vi "ERROR_TEST_MESSAGE.vi"(8 "error in":errorcluster) -> (0 "error out":errorcluster)   [LabVIEW 2012]
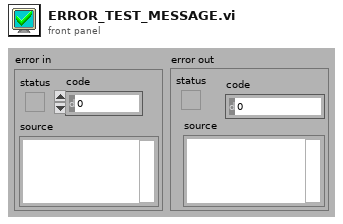
[diagram p1: front panel]
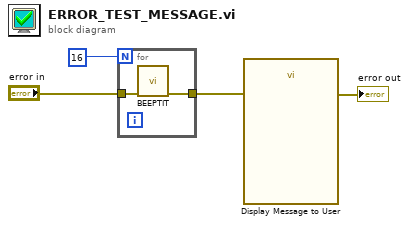
[diagram p0: block diagram]
diagram:
  n1 = for {
    N: 16 -> [_]
    tunnel: "error in" -> [w6]
    tunnel: [w5] -> w2
    n2 = call "BEEPTIT.vi"("error in"=w6) -> ("error out"=w5:errorcluster)  [unwired: 10 in]
  }
  n3 = call "Display Message to User"("error in (no error)"=w2) -> ("error out"=→"error out":errorcluster)  [unwired: 9 in, 1 out]
